vi "dpu_data_read_sa.vi"(8 "error in":errorcluster, 11 "master":refnum<class "Modbus Master.lvclass">) -> (0 "error out":errorcluster, 1 "time":timestamp, 2 "DPU_DATA":T1 {"REL_TREND" format="%#_5e"}, 3 "master":refnum<class "Modbus Master.lvclass">)   [LabVIEW 2014]
uses:
  protocol/modbus/ni_modbus_api/API/Master/Modbus Master.lvclass
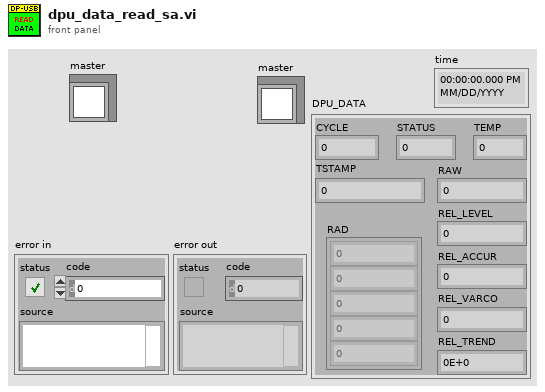
[diagram p1: front panel]
types:
  T1 = cluster{"RAW":i32, "CYCLE":u16, "STATUS":u16, "TSTAMP":u32, "RAD":sgl[], "TEMP":sgl, "REL_LEVEL":sgl, "REL_ACCUR":sgl, "REL_VARCO":sgl, "REL_TREND":sgl}
  T2 = cluster{"register values[0]":u16, "register values[1]":u16, "register values[2]":u16, "register values[3]":u16, "register values[4]":u16, "register values[5]":u16}
  T3 = cluster{"VAL_sgl[0]":sgl, "VAL_sgl[1]":sgl, "VAL_sgl[2]":sgl, "VAL_sgl[3]":sgl}
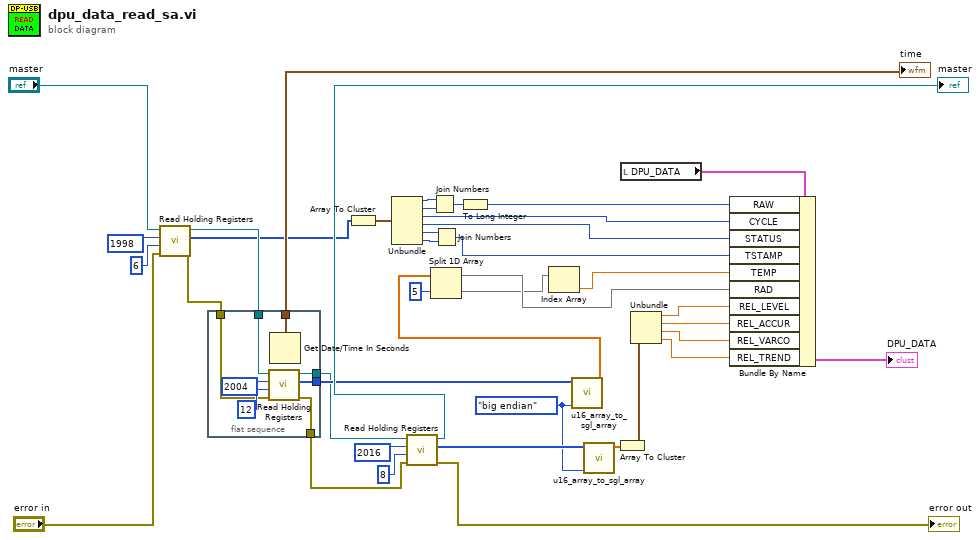
[diagram p0: block diagram]
diagram:
  w16 = enum16{"little endian", "big endian"}."big endian" ("word order")
  n1 = call-dynamic "Read Holding Registers.vi"("error in"="error in", "number of inputs"=u16 6 ("Quantity"), "starting address"=u16 1998 ("Starting Address"), "Modbus master in"="master") -> ("error out"=w28:errorcluster, "register values"=w12:u16[], "Modbus master out"=w31:refnum<class "Modbus Master.lvclass">)  [unwired: 5 in]
  n2 = flat-sequence {
    tunnel: w31 -> [w46]
    tunnel: [w45] -> w30
    tunnel: [w44] -> w29
    tunnel: w28 -> [w43]
    tunnel: [w42] -> w27
    tunnel: [w41] -> w36
    frame #0 {
      n3 = call-dynamic "Read Holding Registers.vi"("error in"=w43, "number of inputs"=u16 12 ("Quantity"), "starting address"=u16 2004 ("Starting Address"), "Modbus master in"=w46) -> ("error out"=w42:errorcluster, "register values"=w45:u16[], "Modbus master out"=w44:refnum<class "Modbus Master.lvclass">)  [unwired: 5 in]
      n4 = Get Date/Time In Seconds() -> (seconds since 1Jan1904=w41:timestamp)
    }
  }
  n5 = Array To Cluster(array=w12) -> (cluster=w18:T2)
  n6 = Unbundle(w18) -> ("register values[0]"=w15:u16, "register values[1]"=w14:u16, "register values[2]"=w7:u16, "register values[3]"=w11:u16, "register values[4]"=w10:u16, "register values[5]"=w9:u16)
  n7 = call-dynamic "Read Holding Registers.vi"("error in"=w27, "number of inputs"=u16 8 ("Quantity"), "starting address"=u16 2016 ("Starting Address"), "Modbus master in"=w29) -> ("error out"=→"error out":errorcluster, "register values"=w23:u16[], "Modbus master out"=→"master":refnum<class "Modbus Master.lvclass">)  [unwired: 5 in]
  n8 = Join Numbers(hi=w15, lo=w14) -> ((hi.lo)=w17:u32)
  n9 = Join Numbers(hi=w10, lo=w9) -> ((hi.lo)=w8:u32)
  n10 = To Long Integer(number=w17) -> (32bit integer=w6:i32)
  n11 = call "u16_array_to_sgl_array.vi"("word order"=w16, "Regs_u16"=w30) -> ("VAL_sgl"=w19:sgl[])  [unwired: 9 in]
  n12 = Split 1D Array(array=w19, index=5) -> (first subarray=w5:sgl[], second subarray=w4:sgl[])
  n13 = Index Array(array=w4) -> (element=w13:sgl)  [unwired: 1 in]
  n14 = call "u16_array_to_sgl_array.vi"("word order"=w16, "Regs_u16"=w23) -> ("VAL_sgl"=w22:sgl[])  [unwired: 9 in]
  n15 = Array To Cluster(array=w22) -> (cluster=w21:T3)
  n16 = local read "DPU_DATA"() -> (w32:T1)
  n17 = Unbundle(w21) -> ("VAL_sgl[0]"=w3:sgl, "VAL_sgl[1]"=w20:sgl, "VAL_sgl[2]"=w2:sgl, "VAL_sgl[3]"=w1:sgl)
  n18 = Bundle By Name(cluster=w32, "RAW"=w6, "CYCLE"=w7, "STATUS"=w11, "TSTAMP"=w8, "TEMP"=w13, "RAD"=w5, "REL_LEVEL"=w3, "REL_ACCUR"=w20, "REL_VARCO"=w2, "REL_TREND"=w1) -> (→"DPU_DATA":T1)
  "time" <- w36
